vi "Update Controls.vi"(8 "error in (no error)":errorcluster, 10 "Control Array":string[][](array[string]), 11 "VI in":refnum<class "VI.lvclass">) -> (0 "error out":errorcluster, 3 "VI out":refnum<class "VI.lvclass">)   [LabVIEW 2020, in "VI Properties Editor.lvlib" / "VI.lvclass"]
doc: "Updates all controls in <B>VI in</B> using the data contained within <B>Control Array</B>."
uses:
  VI.lvclass
  VI.lvclass/VI.ctl
  Control/Control.lvclass
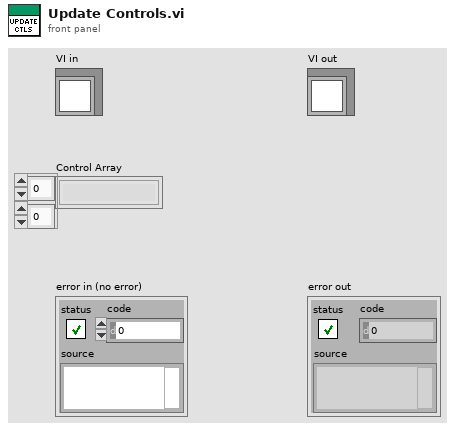
[diagram p1: front panel]
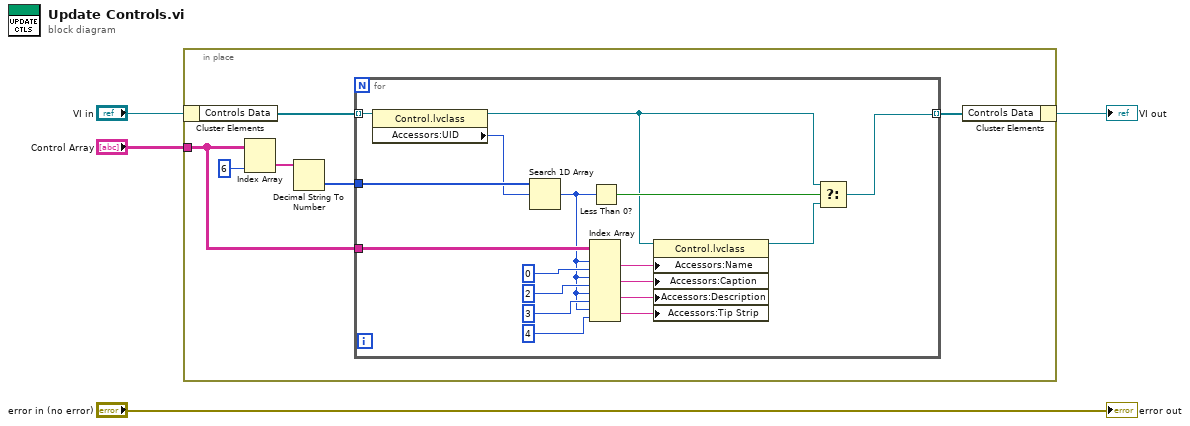
[diagram p0: block diagram]
diagram:
  n1 = in-place {
    in-place-border: "Control Array" -> [w5]
    n2 = in-place-cluster #1("VI in") -> ("Controls Data"=w7:refnum<class "Control.lvclass">[])
    n3 = Index Array(array=w5, index (col)=6 ("disabled index (col)")) -> (element=w9:string[])  [unwired: 1 in]
    n4 = Decimal String To Number(string=w9) -> (number=w10:i32[])  [unwired: 2 in, 1 out]
    n5 = for {
      tunnel: [w21] -> w6 mode=indexing
      tunnel: w7 -> [w13] mode=indexing
      tunnel: w10 -> [w27]
      tunnel: w5 -> [w23]
      n6 = property class="Control.lvclass"(reference=w13) -> (reference out=w11:refnum<class "Control.lvclass">, "Accessors:UID"=w12:i32)  [unwired: 1 in, 1 out]
      n7 = Search 1D Array(1D array=w27, element=w12) -> (index of element=w19:i32)  [unwired: 1 in]
      n8 = Index Array(array=w23, index (row) #1=w19, index (col) #1=0 ("disabled index (col)"), index (row) #2=w19, index (col) #2=2 ("disabled index (col)"), index (row) #3=w19, index (col) #3=3 ("disabled index (col)"), index (row) #4=w19, index (col) #4=4 ("disabled index (col)")) -> (element #1=w17:string, element #2=w16:string, element #3=w15:string, element #4=w14:string)
      n9 = Less Than 0?(x=w19) -> (x < 0?=w22:bool)
      n10 = property class="Control.lvclass"(reference=w11, "Accessors:Name"=w17, "Accessors:Caption"=w16, "Accessors:Description"=w15, "Accessors:Tip Strip"=w14) -> (reference out=w18:refnum<class "Control.lvclass">)  [unwired: 1 in, 1 out]
      n11 = Select(t=w11, s=w22, f=w18) -> (s? t:f=w21:refnum<class "Control.lvclass">)
    }
    n12 = in-place-cluster #1("Controls Data"=w6) -> (→"VI out":refnum<class "VI.lvclass">)
  }
  "error out" <- "error in (no error)"
